vi "BrowerComposite_Create.vi"(6 "SymbolIndex":i32, 8 "error in (no error)":errorcluster, 9 "ComponentName":string, 10 "ComponentID":string, 11 "reference in":refnum<class "BrowerComposite.lvclass">) -> (0 "error out":errorcluster, 3 "reference out":refnum<class "BrowerComposite.lvclass">)   [LabVIEW 2015, in "BrowerComposite.lvclass"]
uses:
  BrowerComposite.lvclass
  BrowerComponent/BrowerComponent.lvclass
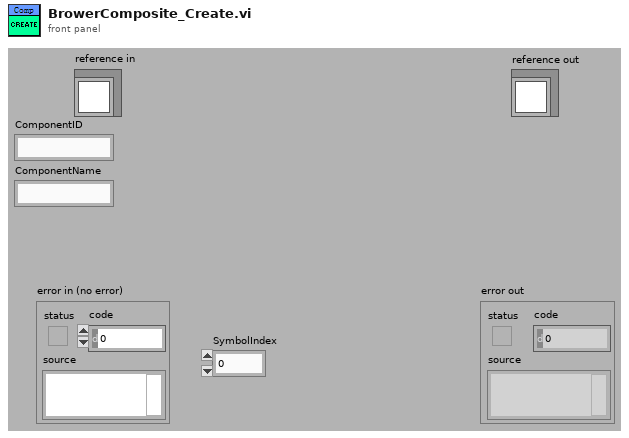
[diagram p1: front panel]
types:
  T1 = typedef "BrowerComposite.lvclass/ObjectAttributes.ctl" = cluster{"BrowerComponents":refnum<class "BrowerComponent.lvclass">[], "BrowerComponentIDs":string[], "Iterator":refnum<class "Iterator.lvclass">}
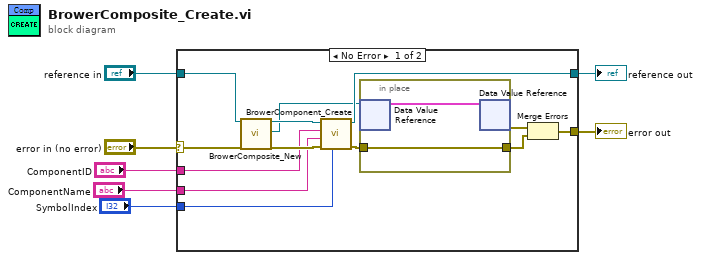
[diagram p0: block diagram]
diagram:
  n1 = case shown="No Error" "error in (no error)" {
    selector: "error in (no error)" -> [w19 w24]
    tunnel: [w17 w24] -> w6
    tunnel: "reference in" -> [w20 w23]
    tunnel: [w14 w23] -> w4
    tunnel: "ComponentID" -> [w10 _]
    tunnel: "ComponentName" -> [w9 _]
    tunnel: "SymbolIndex" -> [w8 _]
    frame No Error {
      n2 = call "BrowerComposite_New.vi"("reference in"=w20, "error in (no error)"=w19) -> ("reference out"=w16:refnum<class "BrowerComposite.lvclass">, "DVRRefOut"=w13:refnum<data-value>, "error out"=w15:errorcluster)  [unwired: 14 in, 1 out]
      n3 = call "BrowerComponent_Create.vi"("SymbolIndex"=w8, "error in (no error)"=w15, "ComponentName"=w9, "ComponentID"=w10, "reference in"=w16) -> ("error out"=w12:errorcluster, "reference out"=w14:refnum<class "BrowerComposite.lvclass">)  [unwired: 5 in]
      n4 = in-place {
        in-place-border: w12 -> [w22]
        in-place-border: [w22] -> w11
        n5 = in-place-dvr #1(w13) -> (w21:T1)  [unwired: 1 out]
        n6 = in-place-dvr #1(w21) -> (w18:errorcluster)  [unwired: 1 out]
      }
      n7 = Merge Errors(w18, w11) -> (w17:errorcluster)
    }
    frame Error {
    }
  }
  "error out" <- w6
  "reference out" <- w4
